vi "Classify Dependencies.vi"(0 "Dependency paths":path[](array[path])) -> (4 "Actual dependencies":path[](array[path]), 6 "DriverVIs":path[](array[path]))   [LabVIEW 2021, in "Multiple Converter.lvlib"]
uses:
  Multiple Converter.lvlib
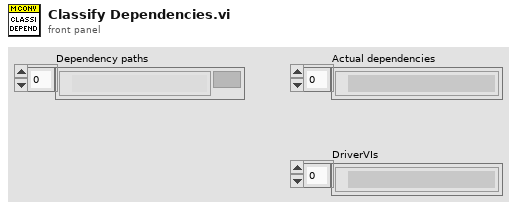
[diagram p1: front panel]
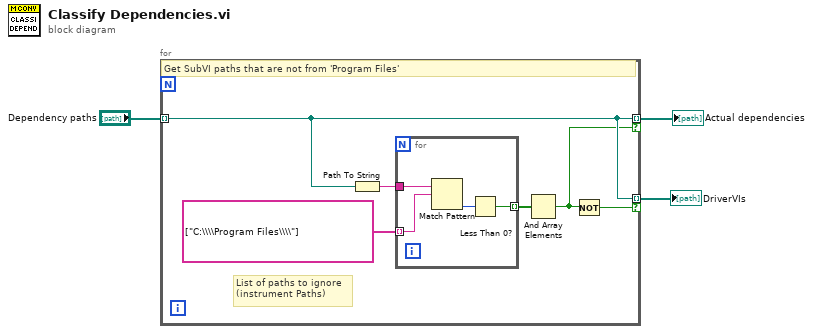
[diagram p0: block diagram]
diagram:
  n1 = for {
    tunnel: "Dependency paths" -> [w8] mode=indexing
    tunnel: [w8] -> w3 mode=indexing if=w5
    tunnel: [w8] -> w1 mode=indexing if=w6
    # "List of paths to ignore\n(instrument Paths)"
    # "Get SubVI paths that are not from 'Program Files'"
    n2 = Path To String(path=w8) -> (string=w9:string)
    n3 = for {
      tunnel: w9 -> [w13]
      tunnel: [w11] -> w7 mode=indexing
      tunnel: string[] ["C:\\\\Program Files\\\\"] -> [w10] mode=indexing
      n4 = Match Pattern(string=w13, regular expression=w10) -> (offset past match=w12:i32)  [unwired: 1 in, 3 out]
      n5 = Less Than 0?(x=w12) -> (x < 0?=w11:bool)
    }
    n6 = And Array Elements(Boolean array=w7) -> (logical AND=w5:bool)
    n7 = Not(x=w5) -> (.not. x?=w6:bool)
  }
  "Actual dependencies" <- w3
  "DriverVIs" <- w1
